vi "Error to Error Response.vi"(9 "error in (no error)":errorcluster) -> (1 "error response":T1)   [LabVIEW 2021]
uses:
  dcvmDPI_AD7606B_server/RPC Messages/dcvmDPI_ErrorResponse.ctl
  dcvmDPI_AD7606B_server/dcvmDPI_AD7606B_server.lvlib
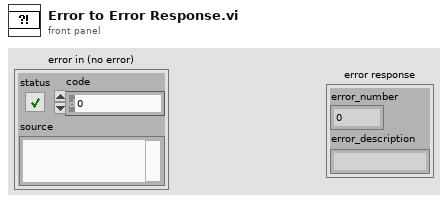
[diagram p1: front panel]
types:
  T1 = typedef "dcvmDPI_AD7606B_server.lvlib/dcvmDPI_ErrorResponse.ctl" = cluster{"error_number":i32, "error_description":string}
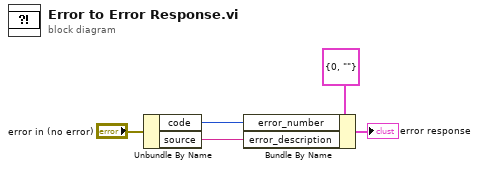
[diagram p0: block diagram]
diagram:
  n1 = Unbundle By Name("error in (no error)") -> ("code"=w2:i32, "source"=w3:string)
  n2 = Bundle By Name(cluster=T1 {"error_number"=0, "error_description"=""} ("dcvmDigitalInterface_ErrorResponse"), "error_number"=w2, "error_description"=w3) -> (→"error response":T1)
